vi "daqio_Connect_User.vi"(6 "daq.io API base":string="http://dashboard.daq.io/api/v1", 7 "Use SSL":bool, 8 "error in (no error)":errorcluster, 9 "timeout for GET routes":i32=10000, 10 "Credentials":T3, 11 "daq.io type in":T1={"daq.io ref"=refnum, "daq.io API Base"="http://dashboard.daq.io/api/v1", "Device Key"="", "Account ID"="", "online"=TRUE, "SSL"=FALSE}) -> (0 "error out":errorcluster, 2 "logged in?":bool, 3 "daq.io type":T1={"daq.io ref"=refnum, "daq.io API Base"="http://dashboard.daq.io/api/v1", "Device Key"="", "Account ID"="", "online"=TRUE, "SSL"=FALSE})   [LabVIEW 2013, in "daqio minimal.lvlib"]
doc: "This VI connects the current user to the daq.io cloud connection."
uses:
  daqio minimal.lvlib
  _typedefs/daqio-Credentials.ctl
  _typedefs/daqio-Type.ctl
  <vilib>/httpClient/ClientHandle.ctl
  _typedefs/daqio-Credentials-FGV.ctl
  <vilib>/httpClient/LabVIEWHTTPClient.lvlib
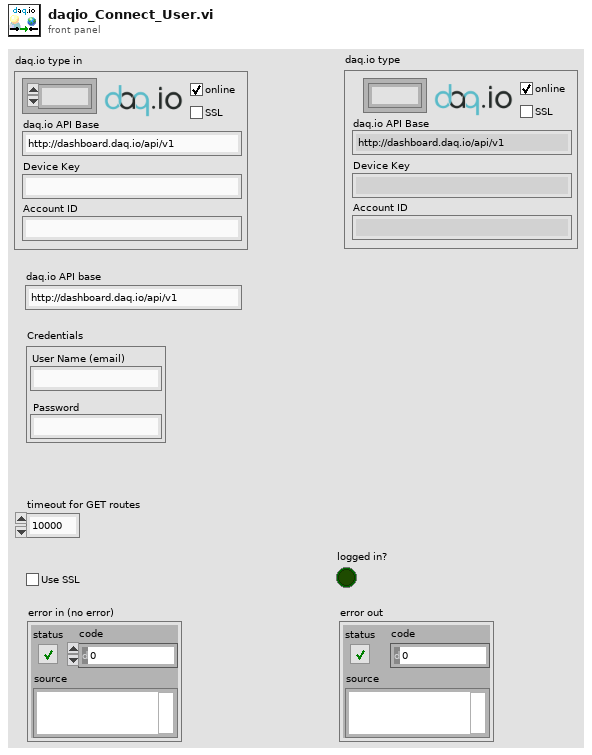
[diagram p1: front panel]
types:
  T1 = typedef "daqio minimal.lvlib/daqio-Type.ctl" = cluster{"daq.io ref":T2, "daq.io API Base":string, "Device Key":string, "Account ID":string, "online":bool, "SSL":bool}
  T2 = typedef "LabVIEWHTTPClient.lvlib/ClientHandle.ctl" = refnum<k1>
  T3 = typedef "daqio minimal.lvlib/daqio-Credentials.ctl" = cluster{"User Name (email)":string, "Password":string}
  T4 = typedef "daqio minimal.lvlib/daqio-Credentials-FGV.ctl" = enum16{"Generate", "Read"}
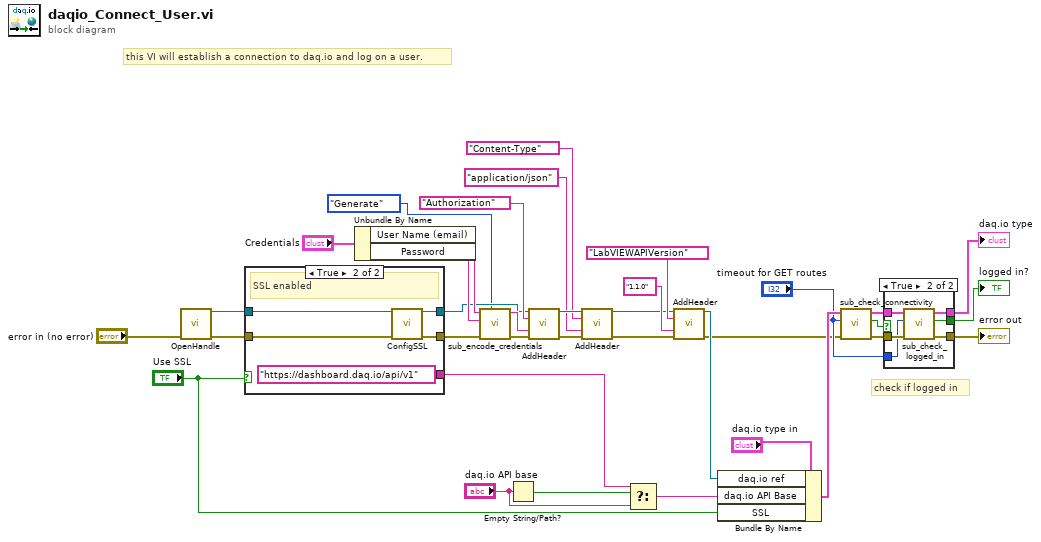
[diagram p0: block diagram]
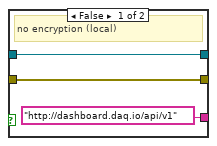
[diagram p2: hidden frame]
diagram:
  # "this VI will establish a connection to daq.io and log on a user."
  # "check if logged in"
  n1 = call <vilib>:"OpenHandle.vi"("error in (no error)"="error in (no error)") -> ("client handle out"=w14:T2, "error out"=w27:errorcluster)  [unwired: 13 in]
  n2 = case shown="True" "Use SSL" {
    tunnel: w27 -> [w38 w44]
    tunnel: [w38 w43] -> w22
    tunnel: [w39 w42] -> w21
    tunnel: w14 -> [w39 w41]
    tunnel: ["http://dashboard.daq.io/api/v1" ("regular API base") "https://dashboard.daq.io/api/v1" ("regular API base")] -> w3
    frame False {
      # "no encryption (local)"
    }
    frame True {
      # "SSL enabled"
      n3 = call <vilib>:"ConfigSSL.vi"("client handle"=w41, "error in (no error)"=w44) -> ("client handle out"=w42:T2, "error out"=w43:errorcluster)  [unwired: 12 in]
    }
  }
  n4 = Unbundle By Name("Credentials") -> ("User Name (email)"=w26:string, "Password"=w25:string)
  n5 = call "sub_encode_credentials.vi"("Command"=daqio-Credentials-FGV."Generate", "error in"=w22, "Password"=w25, "User Name"=w26) -> ("error out"=w23:errorcluster, "Credentials"=w24:string)  [unwired: 5 in, 1 out]
  n6 = Empty String/Path?(string/path="daq.io API base") -> (empty?=w11:bool)
  n7 = call <vilib>:"AddHeader.vi"("client handle"=w21, "header"="Authorization", "value"=w24, "error in (no error)"=w23) -> ("client handle out"=w34:T2, "error out"=w33:errorcluster)  [unwired: 10 in]
  n8 = call <vilib>:"AddHeader.vi"("client handle"=w34, "header"="Content-Type", "value"="application/json", "error in (no error)"=w33) -> ("client handle out"=w28:T2, "error out"=w29:errorcluster)  [unwired: 10 in]
  n9 = Select(t=w3, s=w11, f="daq.io API base") -> (s? t:f=w9:string)
  n10 = call <vilib>:"AddHeader.vi"("client handle"=w28, "header"="LabVIEWAPIVersion", "value"="1.1.0", "error in (no error)"=w29) -> ("client handle out"=w13:T2, "error out"=w6:errorcluster)  [unwired: 10 in]
  n11 = Bundle By Name(cluster="daq.io type in", "daq.io ref"=w13, "daq.io API Base"=w9, "SSL"="Use SSL") -> (w16:T1)
  n12 = call "sub_check_connectivity.vi"("error in (no error)"=w6, "timeout (1000)"="timeout for GET routes", "daq.io type in"=w16) -> ("error out"=w17:errorcluster, "connected"=w15:bool, "daq.io type out"=w18:T1)  [unwired: 6 in]
  n13 = case shown="True" w15 {
    selector: w15 -> [w47 _]
    tunnel: [w45 w53] -> w19
    tunnel: [w47 w52] -> w4
    tunnel: [w46 w51] -> w5
    tunnel: w18 -> [w45 w50]
    tunnel: w17 -> [w46 w49]
    tunnel: "timeout for GET routes" -> [_ w48]
    frame False {
    }
    frame True {
      n14 = call "sub_check_logged_in.vi"("error in (no error)"=w49, "timeout (1000)"=w48, "daq.io type in"=w50) -> ("error out"=w51:errorcluster, "logged in?"=w52:bool, "daq.io type out"=w53:T1)  [unwired: 6 in]
    }
  }
  "error out" <- w5
  "daq.io type" <- w19
  "logged in?" <- w4
